vi "Connection Handler VI.vi"(9 "Additional Data":variant, 10 "connection ID":T1, 11 "TCP Server Refnum":refnum<class "JKI TCP Server.lvclass">) -> ()   [LabVIEW 2020]
uses:
  <vilib>/addons/_JKI.lib/_JKI_lib_TCP_Server.llb/TCP Server Connection Session ID Cluster.ctl
  <vilib>/addons/_JKI.lib/_JKI_lib_TCP_Server.llb/JKI TCP Server.lvclass
  <userlib>/_NEVSTOP/Communicable State Machine(CSM)/_Support/Priority Queue/Priority Queue.lvclass/Priority Queue.ctl
  bd168d05-2ccd-4f69-90c9-be1b4e621865.vi
  316abe05-dd11-44a4-98b3-32ea1594dc48.vi
  a7f8194b-54d4-448d-8a65-d0b66a8fd47c.vi
  8a9da1d4-9237-4126-a3a1-8a9d876b672d.vi
  eb58fbab-51b7-4bfd-aab6-475a21a34b28.vi
  <userlib>/_NEVSTOP/Communicable State Machine(CSM)/_Support/Common/Trim Single line Text.vi
  <userlib>/_NEVSTOP/Communicable State Machine(CSM)/_Support/CSMQ/_Obtain CSM Data Queue.vi
  <userlib>/_NEVSTOP/Communicable State Machine(CSM)/_Support/Priority Queue/Release Priority Queue.vi
  <userlib>/_NEVSTOP/Communicable State Machine(CSM)/AdvanceAPI/CSM - Make String Arguments Safe.vi
  <userlib>/_NEVSTOP/Communicable State Machine(CSM)/_Support/Priority Queue/Obtain Priority Queue.vi
  <userlib>/_NEVSTOP/Communicable State Machine(CSM)/AdvanceAPI/CSM - Keywords.vi
  <userlib>/_NEVSTOP/Communicable State Machine(CSM)/_Support/FGV-BroadcastRegistry/global-CSMQ FGV Change Flag.vi
  <userlib>/_NEVSTOP/Communicable State Machine(CSM)/_Support/CSMQ/_CSMOFGV.vi
  <userlib>/_NEVSTOP/Communicable State Machine(CSM)/addons/API-String-Arugments-Support/_Support/Data To API String Arguments.vi
  <userlib>/_NEVSTOP/Communicable State Machine(CSM)/_Support/Error/CSM No Target Error.vi
  <userlib>/_NEVSTOP/Communicable State Machine(CSM)/_Support/Priority Queue/Priority Queue.lvclass
  <userlib>/_NEVSTOP/Communicable State Machine(CSM)/Communicable State Machine.lvlib
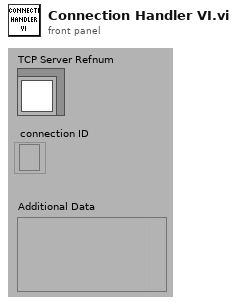
[diagram p1: front panel]
types:
  T1 = typedef "JKI TCP Server.lvclass/TCP Server Connection Session ID Cluster.ctl" = refnum<k5>
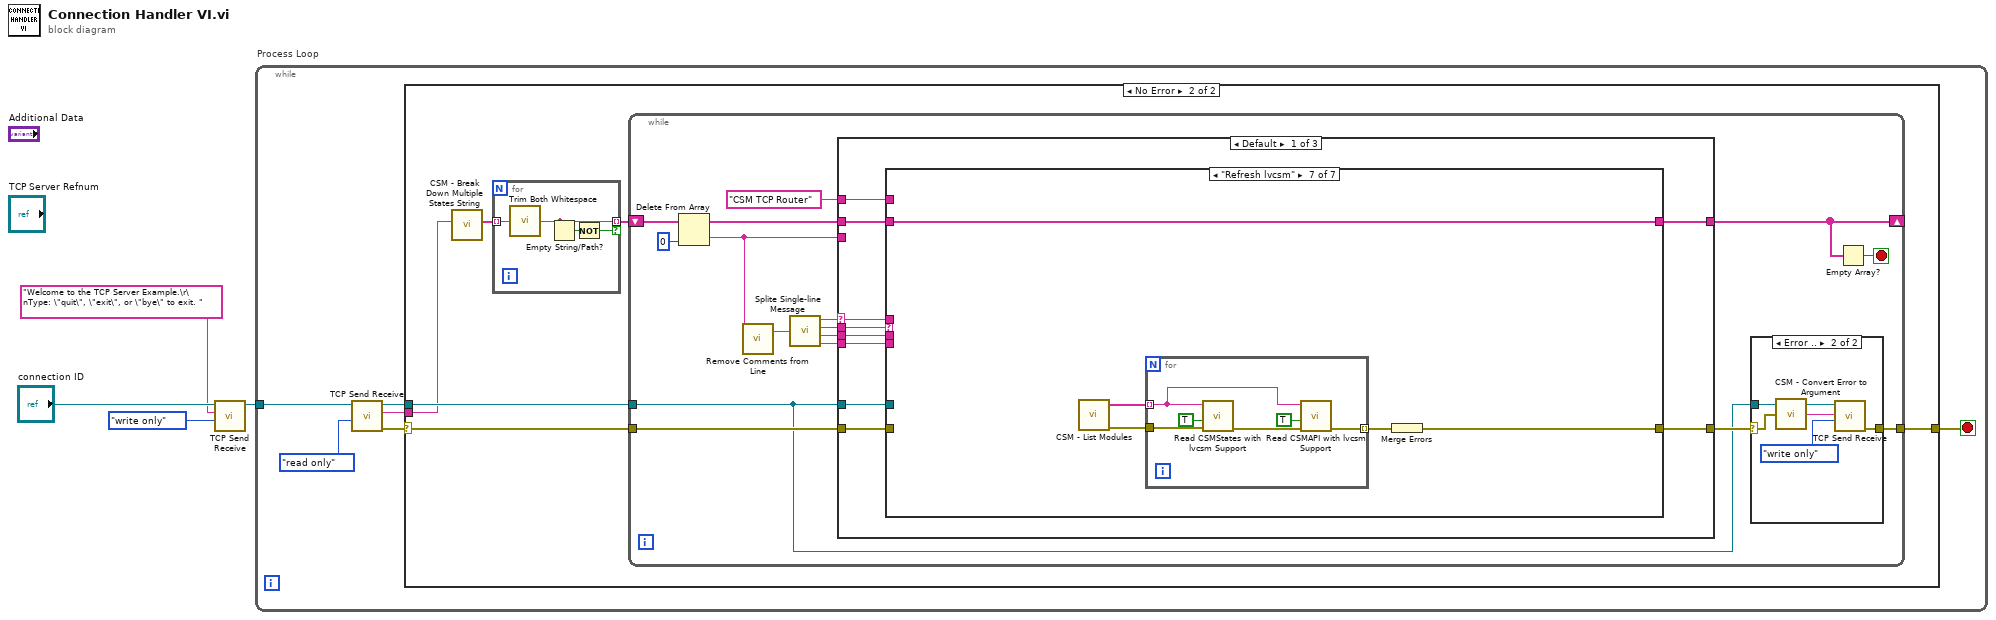
[diagram p0: block diagram]
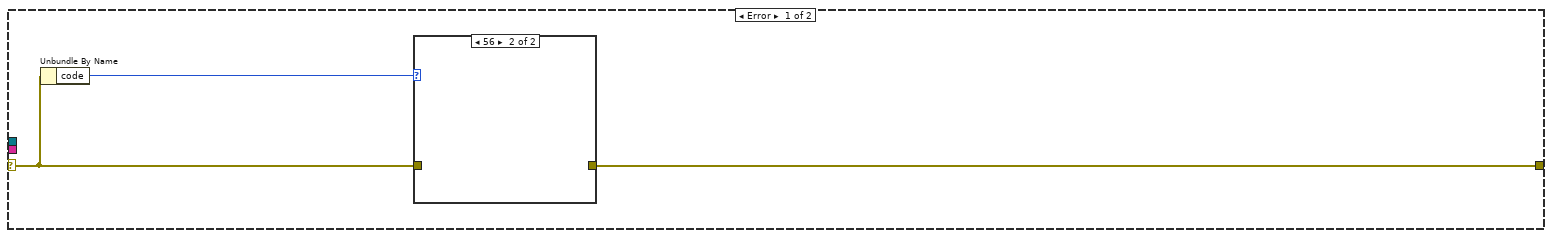
[diagram p2: hidden frame]
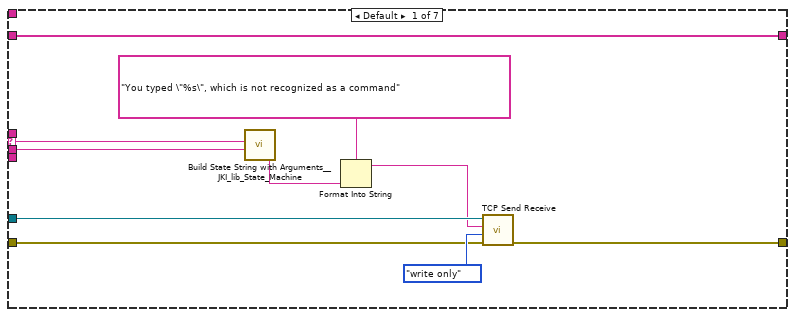
[diagram p5: hidden frame]
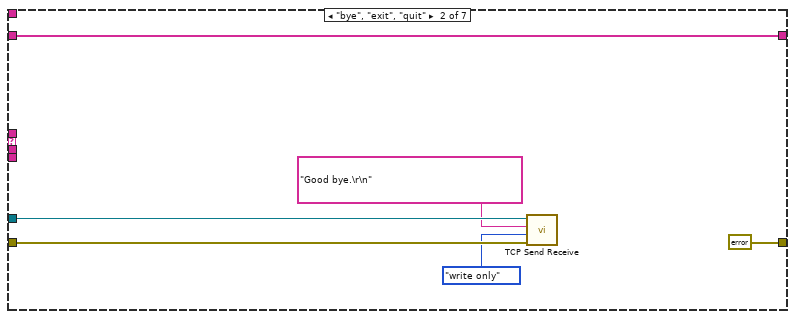
[diagram p6: hidden frame]
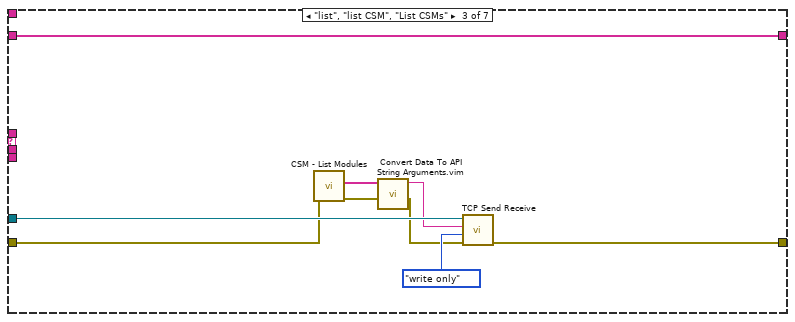
[diagram p7: hidden frame]
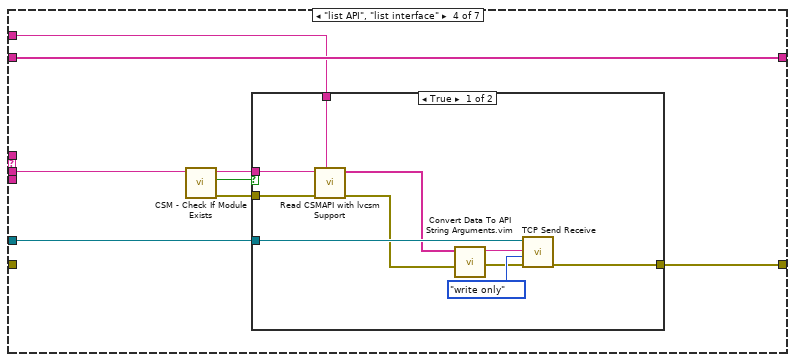
[diagram p8: hidden frame]
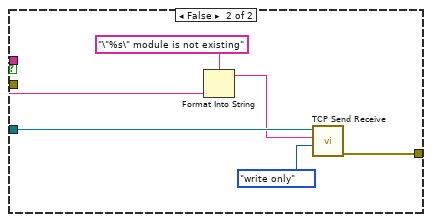
[diagram p9: hidden frame]
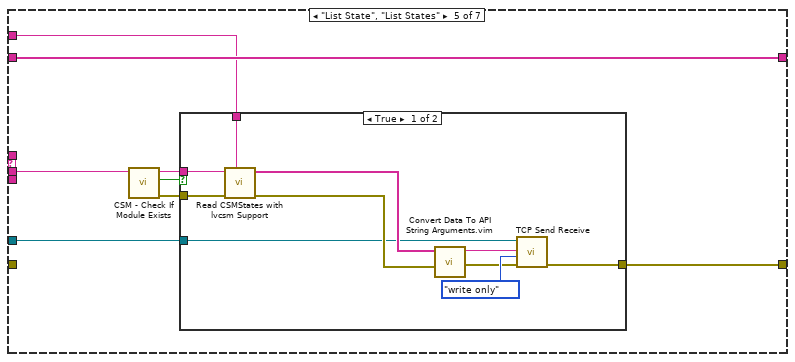
[diagram p10: hidden frame]
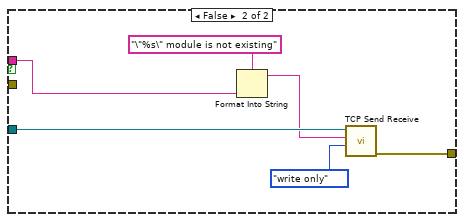
[diagram p11: hidden frame]
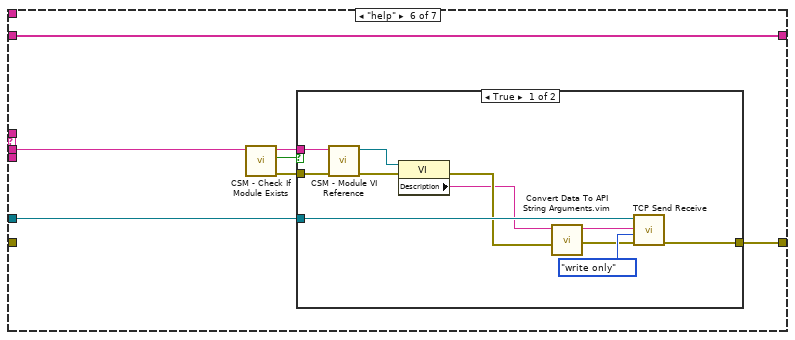
[diagram p12: hidden frame]
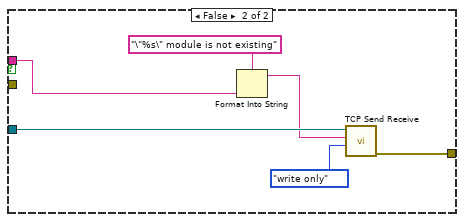
[diagram p13: hidden frame]
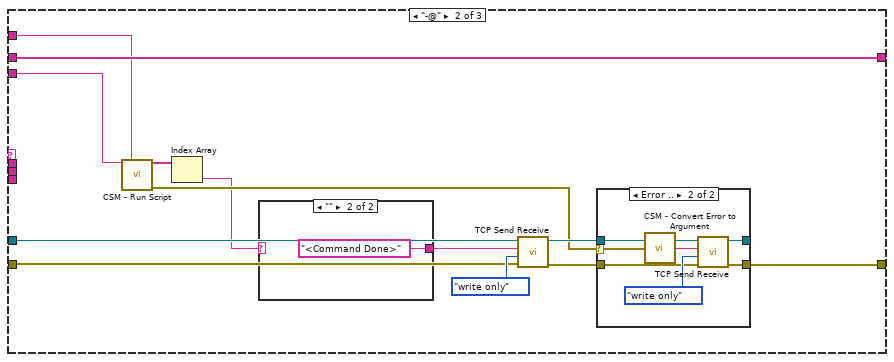
[diagram p14: hidden frame]
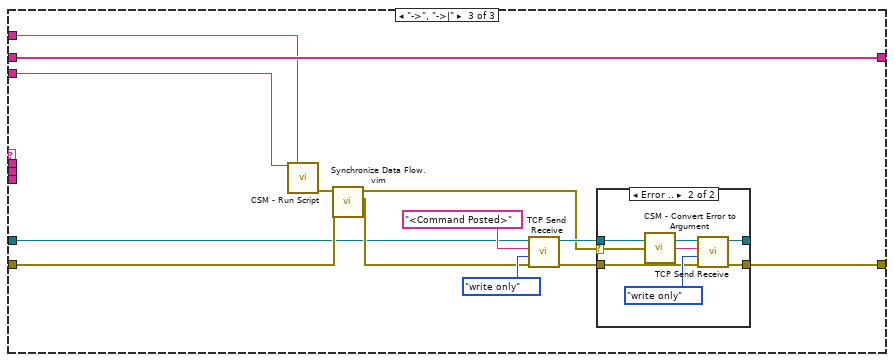
[diagram p17: hidden frame]
diagram:
  n1 = call "TCP Send Receive.vi"("access (read/write)"=enum16{"read/write", "read only", "write only"}."write only", "Data In"="Welcome to the TCP Server Example.\r\nType: \"quit\", \"exit\", or \"bye\" to exit. " ("data in"), "connection ID"="connection ID") -> ("connection ID Out"=w3:refnum<k5>)  [unwired: 6 in, 2 out]
  n2 = while "Process Loop" {
    tunnel: w3 -> [w9]
    stop <- w10 stop-if-true
    n3 = call "TCP Send Receive.vi"("access (read/write)"=enum16{"read/write", "read only", "write only"}."read only", "connection ID"=w9) -> ("error out"=w6:errorcluster, "Data Out"=w5:string, "connection ID Out"=w8:refnum<k5>)  [unwired: 7 in]
    n4 = case shown="No Error" w6 {
      selector: w6 -> [w12 w18]
      tunnel: w8 -> [_ w20]
      tunnel: w5 -> [_ w17]
      tunnel: [w11 w19] -> w10
      frame Error {
        n5 = Unbundle By Name(w12) -> ("code"=w13:i32)
        n6 = case shown="56" w13 {
          tunnel: w12 -> [w14 _]
          tunnel: [w14 _] -> w11
          frame 0, Default {
          }
          frame 56 {
          }
        }
      }
      frame No Error {
        n7 = call <userlib>:"CSM - Break Down Multiple States String.vi"("States"=w17) -> ("Multiple States"=w16:string[])  [unwired: 10 in]
        n8 = for {
          tunnel: w16 -> [w24] mode=indexing
          tunnel: [w23] -> w15 mode=indexing if=w21
          n9 = call <userlib>:"Trim Both Whitespace.vi"("string"=w24) -> ("trimmed string"=w23:string)  [unwired: 1 in]
          n10 = Empty String/Path?(string/path=w23) -> (empty?=w22:bool)
          n11 = Not(x=w22) -> (.not. x?=w21:bool)
        }
        n12 = while {
          tunnel: w20 -> [w27]
          tunnel: w18 -> [w40]
          tunnel: [w28] -> w19
          shift-right: [w30] -> _
          shift-left: w15 -> [w34]
          stop <- w31 stop-if-true
          n13 = Delete From Array(array=w34, index=0) -> (deleted portion=w26:string, array with subset deleted=w33:string[])  [unwired: 1 in]
          n14 = call <userlib>:"Remove Comments from Line.vi"("single-line text"=w26) -> ("single-line text without comments"=w39:string)  [unwired: 2 in]
          n15 = call <userlib>:"Splite Single-line Message.vi"("single-line text"=w39) -> ("operator"=w38:string, "state"=w37:string, "args"=w36:string, "source/target"=w35:string)  [unwired: 6 in]
          n16 = case shown="Default" w38 {
            selector: w38 -> [w50 _ _]
            tunnel: w27 -> [w56 w176 w189]
            tunnel: [w55 w173 w198] -> w29
            tunnel: w40 -> [w54 w169 w195]
            tunnel: w37 -> [w53 _ _]
            tunnel: w36 -> [w52 _ _]
            tunnel: w35 -> [w51 _ _]
            tunnel: [w49 w170 w196] -> w30
            tunnel: w33 -> [w48 w170 w196]
            tunnel: w26 -> [_ w168 w194]
            tunnel: "CSM TCP Router" ("Current Module(\"\" to generate a ID)") -> [w47 w167 w193]
            frame Default {
              n17 = case shown="\"Refresh lvcsm\"" w53 {
                selector: w53 -> [w63 _ _ _ _ _ _]
                tunnel: w56 -> [w66 w70 w81 w89 w113 w136 _]
                tunnel: [w65 errorcluster {"status"=TRUE, "code"=0, "source"=""} ("error out") w74 w88 w112 w135 w154] -> w55
                tunnel: w54 -> [w57 w71 w79 _ _ _ _]
                tunnel: w52 -> [w64 _ _ w84 w108 w131 _]
                tunnel: w51 -> [_ _ _ _ _ _ _]
                tunnel: w50 -> [_ _ _ _ _ _ _]
                tunnel: [w62 w67 w73 w87 w111 w134 w158] -> w49
                tunnel: w48 -> [w62 w67 w73 w87 w111 w134 w158]
                tunnel: w47 -> [_ _ _ w82 w106 _ _]
                frame Default {
                  n18 = call <vilib>:"Build State String with Arguments__JKI_lib_State_Machine.vi"("Arguments (\"\")"=w64, "State"=w63) -> ("State with Arguments"=w58:string)  [unwired: 4 in]
                  n19 = Format Into String(format string="You typed \"%s\", which is not recognized as a command", w58) -> (resulting string=w59:string)  [unwired: 2 in, 1 out]
                  n20 = call "TCP Send Receive.vi"("error in (no error)"=w57, "access (read/write)"=enum16{"read/write", "read only", "write only"}."write only", "Data In"=w59, "connection ID"=w66) -> ("error out"=w65:errorcluster)  [unwired: 5 in, 2 out]
                }
                frame "bye", "exit", "quit" {
                  n21 = call "TCP Send Receive.vi"("error in (no error)"=w71, "access (read/write)"=enum16{"read/write", "read only", "write only"}."write only", "Data In"="Good bye.\r\n" ("data in"), "connection ID"=w70) -> ()  [unwired: 5 in, 3 out]
                }
                frame "list", "list CSM", "List CSMs" {
                  n22 = call <userlib>:"CSM - List Modules.vi"("Error in"=w79) -> ("Error out"=w77:errorcluster, "Module Names"=w78:string[])  [unwired: 9 in]
                  n23 = call "Convert Data To API String Arguments.vim"("error in (no error)"=w77, "data"=w78) -> ("error out"=w76:errorcluster, "String"=w75:string)  [unwired: 6 in]
                  n24 = call "TCP Send Receive.vi"("error in (no error)"=w76, "access (read/write)"=enum16{"read/write", "read only", "write only"}."write only", "Data In"=w75, "connection ID"=w81) -> ("error out"=w74:errorcluster)  [unwired: 5 in, 2 out]
                }
                frame "list API", "list interface" {
                  n25 = call <userlib>:"CSM - Check If Module Exists.vi"("CSM Name"=w84) -> ("Error out"=w86:errorcluster, "Exist?"=w83:bool, "CSM Name(dup)"=w85:string)  [unwired: 8 in]
                  n26 = case shown="True" w83 {
                    tunnel: w89 -> [w99 w105]
                    tunnel: [w98 w104] -> w88
                    tunnel: w86 -> [w94 _]
                    tunnel: w85 -> [w93 w100]
                    tunnel: w82 -> [w90 _]
                    frame True {
                      n27 = call "Read CSMAPI with lvcsm Support.vi"("Current Module(\"\" to generate a ID)"=w90, "error in (no error)"=w94, "CSM Name"=w93) -> ("Error out"=w92:errorcluster, "Value"=w91:string[])  [unwired: 7 in]
                      n28 = call "Convert Data To API String Arguments.vim"("error in (no error)"=w92, "data"=w91) -> ("error out"=w96:errorcluster, "String"=w95:string)  [unwired: 6 in]
                      n29 = call "TCP Send Receive.vi"("error in (no error)"=w96, "access (read/write)"=enum16{"read/write", "read only", "write only"}."write only", "Data In"=w95, "connection ID"=w99) -> ("error out"=w98:errorcluster)  [unwired: 5 in, 2 out]
                    }
                    frame False {
                      n30 = Format Into String(format string="\"%s\" module is not existing", w100) -> (resulting string=w101:string)  [unwired: 2 in, 1 out]
                      n31 = call "TCP Send Receive.vi"("access (read/write)"=enum16{"read/write", "read only", "write only"}."write only", "Data In"=w101, "connection ID"=w105) -> ("error out"=w104:errorcluster)  [unwired: 6 in, 2 out]
                    }
                  }
                }
                frame "List State", "List States" {
                  n32 = call <userlib>:"CSM - Check If Module Exists.vi"("CSM Name"=w108) -> ("Error out"=w110:errorcluster, "Exist?"=w107:bool, "CSM Name(dup)"=w109:string)  [unwired: 8 in]
                  n33 = case shown="True" w107 {
                    tunnel: w113 -> [w115 w129]
                    tunnel: [w123 w128] -> w112
                    tunnel: w110 -> [w118 _]
                    tunnel: w109 -> [w117 w124]
                    tunnel: w106 -> [w114 _]
                    frame True {
                      n34 = call "Read CSMStates with lvcsm Support.vi"("Current Module(\"\" to generate a ID)"=w114, "error in (no error)"=w118, "CSM Name"=w117) -> ("Error out"=w116:errorcluster, "Value"=w119:string[])  [unwired: 7 in]
                      n35 = call "Convert Data To API String Arguments.vim"("error in (no error)"=w116, "data"=w119) -> ("error out"=w121:errorcluster, "String"=w120:string)  [unwired: 6 in]
                      n36 = call "TCP Send Receive.vi"("error in (no error)"=w121, "access (read/write)"=enum16{"read/write", "read only", "write only"}."write only", "Data In"=w120, "connection ID"=w115) -> ("error out"=w123:errorcluster)  [unwired: 5 in, 2 out]
                    }
                    frame False {
                      n37 = Format Into String(format string="\"%s\" module is not existing", w124) -> (resulting string=w125:string)  [unwired: 2 in, 1 out]
                      n38 = call "TCP Send Receive.vi"("access (read/write)"=enum16{"read/write", "read only", "write only"}."write only", "Data In"=w125, "connection ID"=w129) -> ("error out"=w128:errorcluster)  [unwired: 6 in, 2 out]
                    }
                  }
                }
                frame "help" {
                  n39 = call <userlib>:"CSM - Check If Module Exists.vi"("CSM Name"=w131) -> ("Error out"=w133:errorcluster, "Exist?"=w130:bool, "CSM Name(dup)"=w132:string)  [unwired: 8 in]
                  n40 = case shown="True" w130 {
                    tunnel: w136 -> [w140 w153]
                    tunnel: [w147 w152] -> w135
                    tunnel: w133 -> [w143 _]
                    tunnel: w132 -> [w142 w148]
                    frame True {
                      n41 = call <userlib>:"CSM - Module VI Reference.vi"("error in (no error)"=w143, "CSM Name"=w142) -> ("error out"=w141:errorcluster, "CSM Module VIRef"=w138:refnum<vi>)  [unwired: 8 in]
                      n42 = property class="VI"(reference=w138, error in=w141) -> (error out=w139:errorcluster, "Description"=w137:string)  [unwired: 1 out]
                      n43 = call "Convert Data To API String Arguments.vim"("error in (no error)"=w139, "data"=w137) -> ("error out"=w145:errorcluster, "String"=w144:string)  [unwired: 6 in]
                      n44 = call "TCP Send Receive.vi"("error in (no error)"=w145, "access (read/write)"=enum16{"read/write", "read only", "write only"}."write only", "Data In"=w144, "connection ID"=w140) -> ("error out"=w147:errorcluster)  [unwired: 5 in, 2 out]
                    }
                    frame False {
                      n45 = Format Into String(format string="\"%s\" module is not existing", w148) -> (resulting string=w149:string)  [unwired: 2 in, 1 out]
                      n46 = call "TCP Send Receive.vi"("access (read/write)"=enum16{"read/write", "read only", "write only"}."write only", "Data In"=w149, "connection ID"=w153) -> ("error out"=w152:errorcluster)  [unwired: 6 in, 2 out]
                    }
                  }
                }
                frame "Refresh lvcsm" {
                  n47 = call <userlib>:"CSM - List Modules.vi"() -> ("Error out"=w157:errorcluster, "Module Names"=w156:string[])  [unwired: 10 in]
                  n48 = for {
                    tunnel: w157 -> [w164]
                    tunnel: w156 -> [w162] mode=indexing
                    tunnel: [w159] -> w155 mode=indexing
                    n49 = call "Read CSMStates with lvcsm Support.vi"("error in (no error)"=w164, "Force?(F)"=TRUE, "CSM Name"=w162) -> ("Error out"=w163:errorcluster)  [unwired: 7 in, 1 out]
                    n50 = call "Read CSMAPI with lvcsm Support.vi"("error in (no error)"=w163, "Force?(F)"=TRUE, "CSM Name"=w162) -> ("Error out"=w159:errorcluster)  [unwired: 7 in, 1 out]
                  }
                  n51 = Merge Errors(w155) -> (w154:errorcluster)
                }
              }
            }
            frame "-@" {
              n52 = call <userlib>:"CSM - Run Script.vi"("CSM Scripts"=w168, "Current Module(\"\" to generate a ID)"=w167) -> ("Response"=w166:string[], "error out"=w172:errorcluster)  [unwired: 11 in, 1 out]
              n53 = Index Array(array=w166) -> (element=w165:string)  [unwired: 1 in]
              n54 = case shown="\"\"" w165 {
                selector: w165 -> [w178 _]
                tunnel: [w178 "<Command Done>"] -> w171
                frame Default {
                }
                frame "" {
                }
              }
              n55 = call "TCP Send Receive.vi"("error in (no error)"=w169, "access (read/write)"=enum16{"read/write", "read only", "write only"}."write only", "Data In"=w171, "connection ID"=w176) -> ("error out"=w175:errorcluster, "connection ID Out"=w174:refnum<k5>)  [unwired: 5 in, 1 out]
              n56 = case shown="Error .." w172 {
                selector: w172 -> [_ w184]
                tunnel: w175 -> [w181 w187]
                tunnel: w174 -> [w180 w186]
                tunnel: [w181 w185] -> w173
                tunnel: [w180 w182] -> _
                frame No Error {
                }
                frame Error {
                  n57 = call <userlib>:"CSM - Convert Error to Argument.vi"("error"=w184) -> ("Argument"=w183:string)  [unwired: 4 in]
                  n58 = call "TCP Send Receive.vi"("error in (no error)"=w187, "access (read/write)"=enum16{"read/write", "read only", "write only"}."write only", "Data In"=w183, "connection ID"=w186) -> ("error out"=w185:errorcluster, "connection ID Out"=w182:refnum<k5>)  [unwired: 5 in, 1 out]
                }
              }
            }
            frame "->", "->|" {
              n59 = call <userlib>:"CSM - Run Script.vi"("CSM Scripts"=w194, "Current Module(\"\" to generate a ID)"=w193) -> ("error out"=w191:errorcluster)  [unwired: 11 in, 2 out]
              n60 = call "Synchronize Data Flow.vim"("input 2"=w195, "input 1"=w191) -> ("output 2"=w192:errorcluster, "output 1"=w190:errorcluster)  [unwired: 2 in, 2 out]
              n61 = call "TCP Send Receive.vi"("error in (no error)"=w192, "access (read/write)"=enum16{"read/write", "read only", "write only"}."write only", "Data In"="<Command Posted>", "connection ID"=w189) -> ("error out"=w200:errorcluster, "connection ID Out"=w199:refnum<k5>)  [unwired: 5 in, 1 out]
              n62 = case shown="Error .." w190 {
                selector: w190 -> [_ w206]
                tunnel: w200 -> [w203 w209]
                tunnel: w199 -> [w202 w208]
                tunnel: [w203 w207] -> w198
                tunnel: [w202 w204] -> _
                frame No Error {
                }
                frame Error {
                  n63 = call <userlib>:"CSM - Convert Error to Argument.vi"("error"=w206) -> ("Argument"=w205:string)  [unwired: 4 in]
                  n64 = call "TCP Send Receive.vi"("error in (no error)"=w209, "access (read/write)"=enum16{"read/write", "read only", "write only"}."write only", "Data In"=w205, "connection ID"=w208) -> ("error out"=w207:errorcluster, "connection ID Out"=w204:refnum<k5>)  [unwired: 5 in, 1 out]
                }
              }
            }
          }
          n65 = case shown="Error .." w29 {
            selector: w29 -> [w41 w42]
            tunnel: w27 -> [_ w45]
            tunnel: [w41 w44] -> w28
            frame No Error {
            }
            frame Error {
              n66 = call <userlib>:"CSM - Convert Error to Argument.vi"("error"=w42) -> ("Argument"=w43:string)  [unwired: 4 in]
              n67 = call "TCP Send Receive.vi"("access (read/write)"=enum16{"read/write", "read only", "write only"}."write only", "Data In"=w43, "connection ID"=w45) -> ("error out"=w44:errorcluster)  [unwired: 6 in, 2 out]
            }
          }
          n68 = Empty Array?(array=w30) -> (empty?=w31:bool)
        }
      }
    }
  }
